vi "Obtain Main VI Queue.vi"(10 "error in (no error)":errorcluster, 11 "Name (Main VI)":string="Main VI") -> (2 "error out":errorcluster, 3 "queue out":refnum<queue>)   [LabVIEW 2020, in "Dynamic Reentrant.lvlib"]
doc: "Obtains a named queue for the main VI, which has a default name of \"Main VI\" without the quotes. This queue will be created if it does not already exist and uses the Message.ctl typedef to pass data."
uses:
  Dynamic Reentrant.lvlib
  Type Defs/Message.ctl
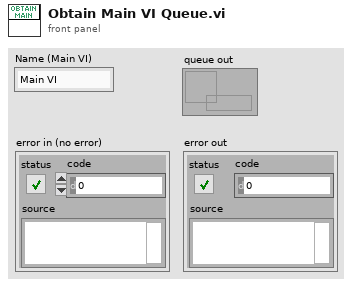
[diagram p1: front panel]
types:
  T1 = typedef "Dynamic Reentrant.lvlib/Message.ctl" = cluster{"Source":string, "Destination":string, "Time Stamp":timestamp, "Command":string, "Data":variant}
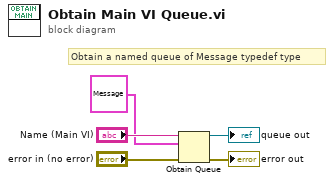
[diagram p0: block diagram]
diagram:
  # "Obtain a named queue of Message typedef type"
  n1 = Obtain Queue(name (unnamed)="Name (Main VI)", element data type=T1 {"Source"="", "Destination"="", "Time Stamp"=timestamp(0 s since 1904-01-01), "Command"="", "Data"=variant(string "")} ("Message"), error in (no error)="error in (no error)") -> (queue out=→"queue out":refnum<queue>, error out=→"error out":errorcluster)  [unwired: 2 in, 1 out]
